vi "UMLEditor_GetNumeric.vi"(8 "error in":errorcluster, 11 "graph":refnum<class "Graph.lvclass">) -> (0 "error out":errorcluster, 3 "Numeric":i16)   [LabVIEW 2016]
uses:
  <resource>/Framework/Providers/Open_GDS/UML/Graph_class/Graph.lvclass
  <resource>/Framework/Providers/Open_GDS/UML/AbstractNode_class/AbstractNode.lvclass
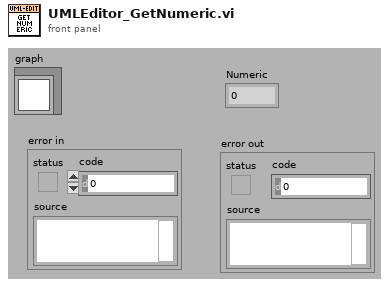
[diagram p1: front panel]
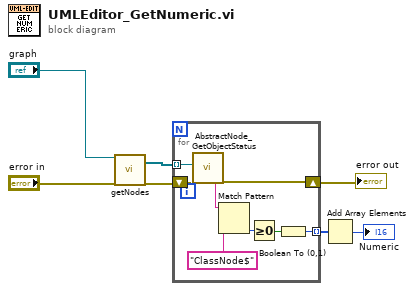
[diagram p0: block diagram]
diagram:
  n1 = call-dynamic "getNodes.vi"("reference"="graph", "error in (no error)"="error in") -> ("nodes"=w5:refnum<class "AbstractNode.lvclass">[], "error out"=w2:errorcluster)  [unwired: 16 out]
  n2 = for {
    shift-right: [w14] -> w1
    shift-left: w2 -> [w15]
    tunnel: w5 -> [w11] mode=indexing
    tunnel: [w8] -> w6 mode=indexing
    n3 = call <resource>:"AbstractNode_GetObjectStatus.vi"("reference in"=w11, "error in (no error)"=w15) -> ("Class name"=w13:string, "error out"=w14:errorcluster)  [unwired: 16 out]
    n4 = Match Pattern(string=w13, regular expression="ClassNode$") -> (offset past match=w10:i32)  [unwired: 4 out]
    n5 = Greater Or Equal To 0?(x=w10) -> (x >= 0?=w9:bool)
    n6 = Boolean To (0,1)(Boolean=w9) -> (0, 1=w8:i16)
  }
  "error out" <- w1
  n7 = Add Array Elements(numeric array=w6) -> (sum=→"Numeric":i16)
